vi "MRC Alert Is Alert Active.vi"(8 "error in (no error)":errorcluster, 11 "handle":i64) -> (0 "error out":errorcluster, 2 "isActive":u8)   [LabVIEW 2026, in "MrcLib.lvlib"]
doc: "MRC_Status MRC_CALLCONV MRC_Alert_IsAlertActive(MRC_AlertHandle handle,\n MRC_Bool* isActive);"
uses:
  MrcLib.lvlib
  MrcLib.dll
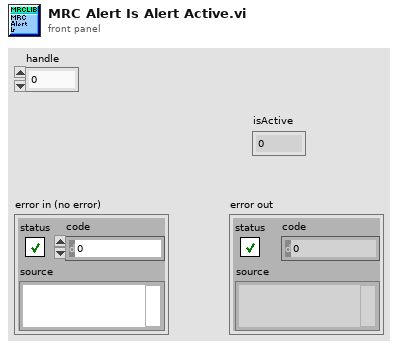
[diagram p1: front panel]
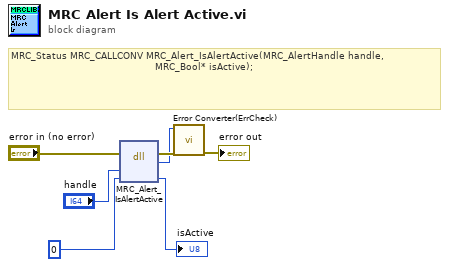
[diagram p0: block diagram]
diagram:
  # "MRC_Status MRC_CALLCONV MRC_Alert_IsAlertActive(MRC_AlertHandle handle,\n                                                MRC_Bool* isActive);"
  n1 = dll-call lib="MrcLib.*" fn="MRC_Alert_IsAlertActive"(error in="error in (no error)", "handle"="handle", "isActive"=u8 0) -> (error out=w3:errorcluster, "return type"=w1:i32, "isActive"=→"isActive":u8)  [unwired: 3 in, 1 out]
  n2 = call <vilib>:"Error Converter(ErrCheck).vi"("error in (no error)"=w3, "status"=w1) -> ("error out"=→"error out":errorcluster)  [unwired: 9 in]
